vi "After Close.vi"(8 "error in":errorcluster, 9 "State In":variant, 10 "Compiled Settings":variant, 11 "Custom Device API in":refnum<class "Custom Device API.lvclass">) -> (0 "error out":errorcluster, 1 "State Out":variant, 3 "Custom Device API out":refnum<class "Custom Device API.lvclass">)   [LabVIEW 2026, in "NIDMM Test Hooks.lvlib"]
uses:
  NIDMM Test Hooks.lvlib
  <userlib>/Custom Device Interfaces_v1.lvlibp/CustomDeviceAPI/Custom Device API.lvclass
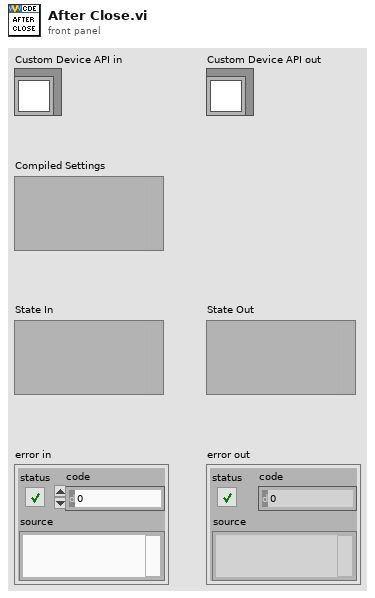
[diagram p1: front panel]
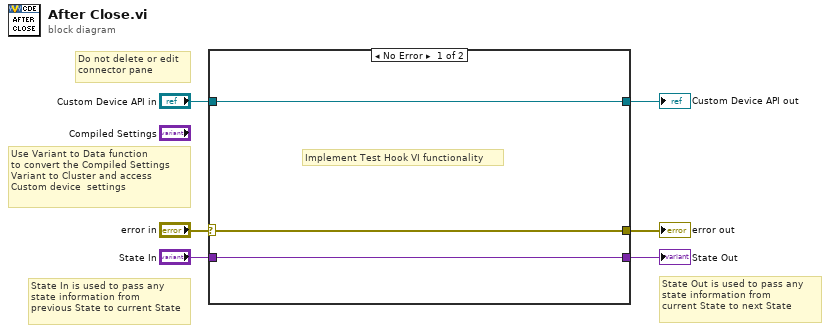
[diagram p0: block diagram]
diagram:
  # "Use Variant to Data function\nto convert the Compiled Settings\nVariant to Cluster and access \nCustom device  settings"
  # "State Out is used to pass any \nstate information from\ncurrent State to next State"
  # "State In is used to pass any \nstate information from\nprevious State to current State"
  # "Do not delete or edit \nconnector pane"
  n1 = case shown="No Error" "error in" {
    selector: "error in" -> [w9 w11]
    tunnel: [w9 w11] -> w5
    tunnel: "Custom Device API in" -> [w8 w12]
    tunnel: [w8 w12] -> w3
    tunnel: "State In" -> [w7 w10]
    tunnel: [w7 w10] -> w1
    frame No Error {
      # "Implement Test Hook VI functionality"
    }
    frame Error {
    }
  }
  "Custom Device API out" <- w3
  "error out" <- w5
  "State Out" <- w1
